vi "Sequencer Main - Copy.vi"() -> ()   [LabVIEW 2018] (continued)
                          n2869 = Array Subset(array=w5897, index=0, length=7) -> (w5898:string[])
                          n2870 = Bundle By Name(cluster=T15 {"Row"=0, "Column"=0} ("Active Cell:Active Cell"), "Row"=w5902, "Column"=5) -> (w5903:T15)
                          n2871 = Replace Array Subset(array=w5910, new element=w5898, index (row)=w5902) -> (w5909:string[][])  [unwired: 1 in]
                          n2872 = property on="Test Sequencer Run" class="MCListbox (strict)"("ItemNames"=w5909, "Value"=w5902, "ActiveCell"=w5903, "CellFontColor"=w5900) -> ()  [unwired: 2 in, 2 out]
                        }
                      }
                    }
                  }
                }
                frame #3 {
                  # "Test Steps Manager"
                  n2873 = in-place {
                    w5928 = 20
                    w5931 = 20
                    n2874 = global read "Global Variable.vi" "Current Step Nmb"() -> (w5935:u32)
                    n2875 = global read "Global Variable.vi" "Report Step Nmb"() -> (w5924:u32)
                    n2876 = Quotient & Remainder(x=w5935, y=w5931) -> (floor(x/y)=w5932:u32)  [unwired: 1 out]
                    n2877 = Quotient & Remainder(x=w5924, y=w5928) -> (floor(x/y)=w5927:u32)  [unwired: 1 out]
                    n2878 = Multiply(x=w5932, y=w5931) -> (x*y=w5930:u32)
                    n2879 = Multiply(x=w5927, y=w5928) -> (x*y=w5929:u32)
                    n2880 = Bundle By Name(cluster=T14 {"Row"=0, "Column"=0} ("Top Left Visible Cell"), "Row"=w5930) -> (w5934:T14)
                    n2881 = Bundle By Name(cluster=T14 {"Row"=0, "Column"=0} ("Top Left Visible Cell"), "Row"=w5929) -> (w5925:T14)
                    n2882 = property on="Test Sequencer" class="MCListbox (strict)"("TopLeft"=w5934) -> ()  [unwired: 2 in, 2 out]
                    n2883 = property on="Test Sequencer Run" class="MCListbox (strict)"("TopLeft"=w5925) -> ()  [unwired: 2 in, 2 out]
                  }
                  n2884 = global read "Global Variable.vi" "Current Step Nmb"() -> (w5920:u32)
                  n2885 = global read "Global Variable.vi" "Steps Nmb"() -> (w5921:u32)
                  n2886 = in-place {
                    n2887 = local read "Tab Edit/Run"() -> (w5936:enum32{"Edit", "Run"})
                    n2888 = case shown="\"Edit\", Default" w5936 {
                      frame "Edit", Default {
                        n2889 = case shown="True" "Delay 1S" {
                          frame False {
                          }
                          frame True {
                            n2890 = Wait (ms)(milliseconds to wait=u32 1000) -> ()  [unwired: 1 out]
                          }
                        }
                      }
                      frame "Run" {
                      }
                    }
                  }
                  n2891 = in-place {
                    # "Prevent False durring run in RUN windows"
                    n2892 = local read "Tab Edit/Run"() -> (w5922:enum32{"Edit", "Run"})
                    n2893 = case shown="\"Run\"" w5922 {
                      frame "Edit", Default {
                      }
                      frame "Run" {
                        n2894 = Wait (ms)(milliseconds to wait=u32 100) -> ()  [unwired: 1 out]
                      }
                    }
                  }
                  n2895 = Decrement(x=w5921) -> (x-1=w5919:u32)
                  n2896 = Equal?(x=w5919, y=w5920) -> (x = y?=w5918:bool)
                  n2897 = case shown="True" w5918 {
                    frame False {
                      n2898 = global write "Global Variable.vi" "System Status"(T1."Run Sequencer" ("System Status")) -> ()
                    }
                    frame True {
                      n2899 = global write "Global Variable.vi" "System Status"(T1."STOP Sequencer" ("System Status")) -> ()
                    }
                  }
                  n2900 = in-place {
                    n2901 = Tick Count (ms)() -> (millisecond timer value=w5939:u32)
                    n2902 = global write "Global Variable.vi" "Test Stop Time"(w5939) -> ()
                  }
                }
              }
            }
          }
        }
        frame "STOP Sequencer" {
          n2903 = in-place {
            in-place-border: w5943 -> [w5945]
            in-place-border: w5942 -> [w5944]
            n2904 = flat-sequence {
              tunnel: w5945 -> [w5993]
              tunnel: w5944 -> [w5992]
              frame #0 {
                n2905 = global read "Global Variable.vi" "Test Gen Status"() -> (w5946:bool)
                n2906 = in-place {
                  # "Create Log File"
                  n2907 = call "Ini_LogFile.vi"() -> ("error out"=w5948:errorcluster, "logFile Path"=w5949:refnum<file>)  [unwired: 10 in]
                  n2908 = global write "Global Variable.vi" "logFile Path"(w5949) -> ()
                  n2909 = local read "LogMsg"() -> (w5953:string)
                  n2910 = Write to Text File(file (use dialog)=w5949, text=w5953, error in=w5948) -> (refnum out=w5951:refnum<file>, error out=w5952:errorcluster)  [unwired: 1 in, 1 out]
                  n2911 = Close File(refnum=w5951, error in=w5952) -> (error out=w5950:errorcluster)  [unwired: 1 out]
                  n2912 = call <userlib>:"Clear All Errors__ogtk.vi"("Error In"=w5950) -> ()  [unwired: 3 in, 1 out]
                }
                n2913 = case shown="True" w5946 {
                  frame False {
                    w5964 = u32 16711680
                    n2914 = Bundle(w5964, w5964) -> (w5965:cluster{u32, u32})  [unwired: 1 in]
                    n2915 = Build Array(w5965) -> (w5966:cluster{u32, u32}[])
                    n2916 = property on="Gen Test Status" class="Bool (strict)"("Colors [4]"=w5966, "Value"=FALSE ("Gen Test Status"), "Strings [4]"=string[] ["FALSE", "PASS", "", ""]) -> ()  [unwired: 2 in, 2 out]
                  }
                  frame True {
                    w5969 = u32 40735
                    n2917 = Bundle(w5969, w5969) -> (w5967:cluster{u32, u32})  [unwired: 1 in]
                    n2918 = Build Array(w5967) -> (w5968:cluster{u32, u32}[])
                    n2919 = property on="Gen Test Status" class="Bool (strict)"("Colors [4]"=w5968, "Value"=TRUE ("Gen Test Status"), "Strings [4]"=string[] ["FALSE", "PASS", "", ""]) -> ()  [unwired: 2 in, 2 out]
                  }
                }
                n2920 = case shown="True" FALSE {
                  frame False {
                  }
                  frame True {
                    n2921 = One Button Dialog(message="STOP Sequencer") -> ()  [unwired: 1 in, 1 out]
                  }
                }
                n2922 = in-place {
                  in-place-border: w5946 -> [w5954]
                  n2923 = local read "Cnt Total"() -> (w5955:i32)
                  n2924 = case shown="True" w5954 {
                    frame False {
                      n2925 = local read "Cnt False"() -> (w5958:i32)
                      n2926 = Increment(x=w5958) -> (x+1=w5957:i32)
                      n2927 = local write "Cnt False"(w5957) -> ()
                    }
                    frame True {
                      n2928 = local read "Cnt Pass"() -> (w5960:i32)
                      n2929 = Increment(x=w5960) -> (x+1=w5959:i32)
                      n2930 = local write "Cnt Pass"(w5959) -> ()
                    }
                  }
                  n2931 = Increment(x=w5955) -> (x+1=w5956:i32)
                  n2932 = local write "Cnt Total"(w5956) -> ()
                }
              }
              frame #1 {
                w5974 = FALSE ("Enable Output")
                w5972 = 0.1 ("Current")
                w5973 = 0.0 ("Voltage")
                n2933 = global read "Global Variable.vi" "VISA Resource Name BK-9202"() -> (w5983:string)
                n2934 = call "bk9201 Set.vi"("Enable Output"=w5974, "Current"=w5972, "Voltage"=w5973, "VISA resource name"=w5983) -> ("error out"=w5979:errorcluster)  [unwired: 7 in]
                n2935 = local read "PowSupply - SET"() -> (w5976:T7)
                n2936 = local read "Switch Relay Modules"() -> (w5978:T5)
                n2937 = Bundle By Name(cluster=w5978, "Main Power Supplay ON/OFF"=w5974) -> (w5977:T5)
                n2938 = global read "Global Variable.vi" "Array Errors"() -> (w5981:errorcluster[])
                n2939 = Bundle By Name(cluster=w5976, "ON/OFF"=w5974, "Volt (V)"=w5973, "Current Limit (A)"=w5972) -> (w5975:T7)
                n2940 = global write "Global Variable.vi" "PowSupply ON/OFF"(w5974) -> ()
                n2941 = Replace Array Subset(array=w5981, new element=w5979, index=2) -> (w5982:errorcluster[])
                n2942 = local write "Switch Relay Modules"(w5977) -> ()
                n2943 = local write "PowSupply - SET"(w5975) -> ()
                n2944 = global write "Global Variable.vi" "Array Errors"(w5982) -> ()
              }
              frame #2 {
                n2945 = global read "Global Variable.vi" "COM Port RFID"() -> (w5987:refnum<visa-resource-name>)
                n2946 = call "Stop Reading.vi"("error in (no error)"=errorcluster {"status"=FALSE, "code"=0, "source"=""}, "Baud Rate"=u32 38400, "COM Port"=w5987) -> ("error out"=w5984:errorcluster)  [unwired: 6 in, 2 out]
                n2947 = call <userlib>:"Clear All Errors__ogtk.vi"("Error In"=w5984) -> ()  [unwired: 3 in, 1 out]
              }
              frame #3 {
                n2948 = call <vilib>:"Acquire Semaphore.vi"("error in (no error)"=w5993, "semaphore"=w5992) -> ("error out"=w5991:errorcluster, "semaphore out"=w5990:T13)  [unwired: 3 in, 1 out]
                n2949 = case shown="No Error" w5991 {
                  selector: w5991 -> [w6005 w6052]
                  tunnel: w5990 -> [w6004 w6051]
                  tunnel: [w6005 w6052] -> w5989
                  tunnel: [w6004 w6051] -> w5988
                  frame No Error {
                    w5999 = u8 1  # nCS
                    w6000 = T20 0 items=["Addr-0"=0, "Addr-1"=4, "Addr-2"=2, "Addr-3"=6, "Addr-4"=1, "Addr-5"=5, "Addr-6"=3, "Addr-7"=7] ("Addr")
                    w6010 = T20 7 items=["Addr-0"=0, "Addr-1"=4, "Addr-2"=2, "Addr-3"=6, "Addr-4"=1, "Addr-5"=5, "Addr-6"=3, "Addr-7"=7] ("Addr")
                    # "FALSE"
                    # "PASS"
                    # "nCS"
                    n2950 = global read "Global Variable.vi" "FTDI SPI Handle"() -> (w6001:u32)
                    n2951 = for {
                      N: 4 -> [_]
                      tunnel: w6001 -> [w6029]
                      tunnel: [w6021] -> w6011
                      i -> [w6024]
                      w6026 = u8 0  # nCS
                      w6025 = u16 0  # Channel Decimal
                      w6027 = TRUE  # Use Extra
                      n2952 = call "FTDI SPI GPIO Set.vi"("nCS"=w6026, "Mode"=T23."Set Decimal", "Use Extra"=w6027, "Channel Decimal"=w6025, "Addr"=w6024, "Handler In"=w6029) -> ("error out"=w6021:errorcluster, "LATCH Reg"=w6022:u16)  [unwired: 2 in, 2 out]
                      n2953 = Number To Boolean Array(number=w6022) -> (Boolean array=w6023:bool[])
                      n2954 = case shown="0" w6024 {
                        tunnel: w6023 -> [_ w6030 w6033 w6036 w6039 w6042 w6045 w6048]
                        frame -1, Default {
                        }
                        frame 0 {
                          n2955 = local read "Switch Relay Modules"() -> (w6032:T5)
                          n2956 = Bundle By Name(cluster=w6032, "SW 0"=w6030) -> (w6031:T5)
                          n2957 = local write "Switch Relay Modules"(w6031) -> ()
                        }
                        frame 1 {
                          n2958 = local read "Switch Relay Modules"() -> (w6035:T5)
                          n2959 = Bundle By Name(cluster=w6035, "SW 1"=w6033) -> (w6034:T5)
                          n2960 = local write "Switch Relay Modules"(w6034) -> ()
                        }
                        frame 2 {
                          n2961 = local read "Switch Relay Modules"() -> (w6038:T5)
                          n2962 = Bundle By Name(cluster=w6038, "SW 2"=w6036) -> (w6037:T5)
                          n2963 = local write "Switch Relay Modules"(w6037) -> ()
                        }
                        frame 3 {
                          n2964 = local read "Switch Relay Modules"() -> (w6041:T5)
                          n2965 = Bundle By Name(cluster=w6041, "SW 3"=w6039) -> (w6040:T5)
                          n2966 = local write "Switch Relay Modules"(w6040) -> ()
                        }
                        frame 4 {
                          n2967 = local read "Switch Relay Modules"() -> (w6044:T5)
                          n2968 = Bundle By Name(cluster=w6044, "SW 4"=w6042) -> (w6043:T5)
                          n2969 = local write "Switch Relay Modules"(w6043) -> ()
                        }
                        frame 5 {
                          n2970 = local read "Switch Relay Modules"() -> (w6047:T5)
                          n2971 = Bundle By Name(cluster=w6047, "SW 5"=w6045) -> (w6046:T5)
                          n2972 = local write "Switch Relay Modules"(w6046) -> ()
                        }
                        frame 6 {
                          n2973 = local read "Switch Relay Modules"() -> (w6050:T5)
                          n2974 = Bundle By Name(cluster=w6050, "SW 6"=w6048) -> (w6049:T5)
                          n2975 = local write "Switch Relay Modules"(w6049) -> ()
                        }
                      }
                    }
                    n2976 = local read "Gen Test Status"() -> (w5996:bool)
                    n2977 = global read "Global Variable.vi" "FTDI SPI Handle"() -> (w6016:u32)
                    n2978 = Select(t=1, s=w5996, f=2) -> (s? t:f=w5997:i32)
                    n2979 = call "FTDI SPI GPIO Set.vi"("nCS"=u8 2, "Mode"=T24."Set Decimal", "Use Extra"=TRUE, "Channel Decimal"=w5997, "Addr"=w6010, "Handler In"=w6016) -> ("error out"=w6012:errorcluster, "LATCH Reg"=w6009:u16)  [unwired: 2 in, 2 out]
                    n2980 = local read "Switch Relay Modules"() -> (w6007:T5)
                    n2981 = Number To Boolean Array(number=w6009) -> (Boolean array=w6008:bool[])
                    n2982 = Bundle By Name(cluster=w6007, "SW 7"=w6008) -> (w6006:T5)
                    n2983 = global read "Global Variable.vi" "Array Errors"() -> (w6019:errorcluster[])
                    n2984 = Merge Errors(w6011, w6012) -> (w6013:errorcluster)
                    n2985 = local write "Switch Relay Modules"(w6006) -> ()
                    n2986 = Replace Array Subset(array=w6019, new element=w6013, index=10) -> (w6020:errorcluster[])
                    n2987 = call "FTDI SPI GPIO Set.vi"("nCS"=w5999, "Use Extra"=TRUE, "Channel Decimal"=u16 0, "Addr"=w6000, "Handler In"=w6001) -> ()  [unwired: 3 in, 4 out]
                    n2988 = global write "Global Variable.vi" "Array Errors"(w6020) -> ()
                  }
                  frame Error {
                  }
                }
                n2989 = call <vilib>:"Release Semaphore.vi"("error in (no error)"=w5989, "semaphore"=w5988) -> ()  [unwired: 4 in, 2 out]
              }
              frame #4 {
                n2990 = local read "Restart Cnt"() -> (w6054:u16)
                n2991 = local read "Auto\nRestart"() -> (w6055:u16)
                n2992 = Less?(x=w6054, y=w6055) -> (x < y?=w6056:bool)
                n2993 = case shown="True" w6056 {
                  frame False {
                    n2994 = local read "Report Auto"() -> (w6060:bool)
                    n2995 = case shown="True" w6060 {
                      frame False {
                        n2996 = global write "Global Variable.vi" "System Status"(T1."Idle" ("System Status")) -> ()
                      }
                      frame True {
                        n2997 = global read "Global Variable.vi" "Retest Nmb"() -> (w6062:i16)
                        n2998 = case shown="0, Default" w6062 {
                          frame 0, Default {
                            n2999 = property on="Tab Control Main" class="TabCtl (strict)"("Value"=T2."Report" ("Tab Control Main")) -> ()  [unwired: 2 in, 2 out]
                            n3000 = global write "Global Variable.vi" "System Status"(T1."Report Generation" ("System Status")) -> ()
                          }
                          frame 1 {
                            n3001 = global write "Global Variable.vi" "Test Gen Status"(FALSE ("Test Gen Status")) -> ()
                            n3002 = global write "Global Variable.vi" "System Status"(T1."Idle" ("System Status")) -> ()
                          }
                        }
                      }
                    }
                    n3003 = local write "Auto\nRestart"(1) -> ()
                    n3004 = local write "Message"(">>>STOP SEQUENSER <<<") -> ()
                    n3005 = property on="Run Test" class="Bool"("DisabledEnum"=T18."Enabled" ("Disabled")) -> ()  [unwired: 2 in, 2 out]
                  }
                  frame True {
                    n3006 = local write "Auto\nReStart"(TRUE ("Auto\nReStart")) -> ()
                    n3007 = global write "Global Variable.vi" "Reset BARCODE"(TRUE ("Reset BARCODE")) -> ()
                    n3008 = local read "Report Auto"() -> (w6068:bool)
                    n3009 = case shown="False" w6068 {
                      frame False {
                        # "Idle"
                        n3010 = global write "Global Variable.vi" "System Status"(T1."Idle" ("System Status")) -> ()
                        n3011 = property on="Tab Control Main" class="TabCtl (strict)"("Value"=T2."TEST Board" ("Tab Control Main")) -> ()  [unwired: 2 in, 2 out]
                      }
                      frame True {
                        n3012 = global write "Global Variable.vi" "System Status"(T1."Report Generation" ("System Status")) -> ()
                        n3013 = property on="Tab Control Main" class="TabCtl (strict)"("Value"=T2."Report" ("Tab Control Main")) -> ()  [unwired: 2 in, 2 out]
                      }
                    }
                    n3014 = local write "Message"(">>> RESTART TEST Sequencer <<<") -> ()
                  }
                }
                n3015 = property on="Msg Str" class="Str"("Value"="STOP SEQUENSER\nReset ALL") -> ()  [unwired: 2 in, 2 out]
              }
            }
          }
        }
        frame "Report Generation" {
          n3016 = flat-sequence {
            tunnel: [w6089] -> w6082
            tunnel: [w6088] -> w6081
            tunnel: [w6085] -> w6080
            tunnel: [w6123] -> w6084
            tunnel: [w6122] -> w6083
            tunnel: w6082 -> [w6122]
            tunnel: w6081 -> [w6121]
            tunnel: w6080 -> [w6119]
            tunnel: w6084 -> [w6133]
            tunnel: [w6132] -> w6079
            tunnel: w6083 -> [w6132]
            tunnel: w6079 -> [w6140]
            tunnel: [w6141] -> w6078
            tunnel: [w6140] -> w6077
            tunnel: [w6138] -> w6076
            tunnel: [w6139] -> w6075
            tunnel: w6078 -> [w6180]
            tunnel: w6077 -> [w6179]
            tunnel: w6076 -> [w6177]
            tunnel: w6075 -> [w6178]
            frame #0 {
              w6086 = "<p>&nbsp;</p>" ("string")
              w6112 = u16 2 items=["Default", "US", "Metric"] ("measurement system (default)")
              # "table {\n  font-family: arial, sans-serif;\n  border-collapse: collapse;\n  width: 70%;\n}"
              # "Hardware Revision"
              n3017 = property on="Test Sequencer Run" class="MCListbox (strict)"() -> ("ColHdrString"=w6118:string[], "ItemNames"=w6114:string[][])  [unwired: 2 in, 2 out]
              n3018 = local read "Test Time"() -> (w6094:string)
              n3019 = call <vilib>:"New Report.vi"("report type"=T31."HTML") -> ("report out"=w6108:refnum<class "NI_report.lvclass">, "error out"=w6111:errorcluster)  [unwired: 5 in, 8 out]
              n3020 = local read "Customer"() -> (w6105:string)
              n3021 = local read "Under Test BOARD"() -> (w6104:string)
              n3022 = local read "Barcode"() -> (w6101:string)
              n3023 = property on="Operator" class="Ring (strict)"() -> ("RingText.Text"=w6100:string)  [unwired: 2 in, 2 out]
              n3024 = local read "Config"() -> (w6103:string)
              n3025 = global read "Global Variable.vi" "Report Step Nmb"() -> (w6091:u32)
              n3026 = call-dynamic "Set Report Margins.vi"("report in"=w6108, "margins (1.00)"=T32 {"top"=10.0, "left"=10.0, "right"=10.0, "bottom"=10.0}, "measurement system (default)"=w6112, "error in (no error)"=w6111) -> ("report out"=w6109:refnum<class "NI_report.lvclass">, "error out"=w6110:errorcluster)  [unwired: 9 in, 1 out]
              n3027 = local read "Gen Test Status"() -> (w6099:bool)
              n3028 = Array Subset(array=w6118, index=0, length=7) -> (w6115:string[])
              n3029 = Concatenate Strings("Measurement Results" ("Table Header"), "    (", "TestTime -" ("Table Header"), w6094, ")") -> (w6096:string)
              n3030 = Increment(x=w6091) -> (x+1=w6090:u32)
              n3031 = Build Array (concatenate)(w6115, w6114) -> (w6113:string[][])
              n3032 = call "html Header.vi"("Test Result"=w6099, "Test Operator"=w6100, "Company"=w6105, "Serial Numbe (SN)"=w6101, "Hardware Revision"="v1.1", "Product Info"=w6103, "Product Name"=w6104) -> ("html string"=w6087:string)  [unwired: 4 in]
              n3033 = call "html Table.vi"("Rows cnt"=w6090, "Table Header"=w6096, "In String Table"=w6113) -> ("html string out"=w6098:string)  [unwired: 8 in]
              n3034 = Concatenate Strings(w6087, w6086, w6098, w6086) -> (w6089:string)
              n3035 = call-dynamic "Append User Formatted HTML to Report.vi"("report in"=w6109, "HTML text"=w6089, "error in (no error)"=w6110) -> ("report out"=w6085:refnum<class "NI_report.lvclass">, "error out"=w6088:errorcluster)  [unwired: 11 out]
            }
            frame #1 {
              n3036 = in-place {
                in-place-border: w6119 -> [w6129]
                in-place-border: [w6128] -> w6123
                # "Local Temp File"
                n3037 = call <vilib>:"Application Directory.vi"() -> ("Application Directory"=w6131:path)
                n3038 = Build Path(base path=w6131, name or relative path="report.html") -> (appended path=w6128:path)
                n3039 = call-dynamic "Save Report to File.vi"("report in"=w6129, "report file path"=w6128) -> ()  [unwired: 12 in, 2 out]
                n3040 = Wait (ms)(milliseconds to wait=u32 250) -> ()  [unwired: 1 out]
              }
              n3041 = case shown="True" "Open in Default IE" {
                tunnel: w6121 -> [_ w6126]
                tunnel: w6119 -> [_ w6125]
                frame False {
                  n3042 = Wait (ms)(milliseconds to wait=u32 2000) -> ()  [unwired: 1 out]
                }
                frame True {
                  # "Open HTML Report in Browser VI"
                  n3043 = call-poly <vilib>:"Open HTML Report in Browser.vi"("report in"=w6125, "error in (no error)"=w6126) -> ()  [unwired: 14 out]
                }
              }
            }
            frame #2 {
              n3044 = Path To String(path=w6133) -> (string=w6136:string)
              n3045 = invoke class="IWebBrowser2" method="Navigate"(reference="WebBrowser", "URL"=w6136) -> (error out=w6134:errorcluster)  [unwired: 6 in, 7 out]
              n3046 = call <userlib>:"Clear All Errors__ogtk.vi"("Error In"=w6134) -> ()  [unwired: 3 in, 1 out]
            }
            frame #3 {
              # "Create BARCODE / Number FOLDER"
              n3047 = global read "Global Variable.vi" "DB Dir Path"() -> (w6137:path)
              n3048 = in-place {
                in-place-border: [w6159] -> w6139
                in-place-border: [w6146] -> w6138
                in-place-border: w6137 -> [w6144]
                # "Sub Dir?"
                # "FALSE Sub Dir?"
                n3049 = Get Date/Time String() -> (date string=w6154:string)  [unwired: 3 in, 1 out]
                n3050 = while {
                  shift-right: [w6170] -> w6155
                  shift-left: w6154 -> [w6173]
                  stop <- w6168 stop-if-true
                  # "Replase character / to _"
                  n3051 = call <vilib>:"Search and Replace Pattern.vi"("string"=w6173, "regular expression (\"\")"="/" ("substring (\"\")"), "replace string (\"\")"="_" ("replace string (\"\")")) -> ("result string"=w6170:string, "offset past match"=w6169:i32)  [unwired: 2 in]
                  n3052 = Less Than 0?(x=w6169) -> (x < 0?=w6168:bool)
                }
                n3053 = local read "Config"() -> (w6148:string)
                n3054 = Build Path(base path=w6144, name or relative path=w6155) -> (appended path=w6149:path)
                n3055 = Build Path(base path=w6149, name or relative path=w6148) -> (appended path=w6147:path)
                n3056 = call <vilib>:"Check if File or Folder Exists.vi"("path"=w6147) -> ("file or folder exists?"=w6153:bool, "dup path"=w6158:path)  [unwired: 8 in, 1 out]
                n3057 = Not(x=w6153) -> (.not. x?=w6157:bool)
                n3058 = case shown="True" w6157 {
                  tunnel: w6158 -> [w6164 w6167]
                  tunnel: [w6164 w6165] -> w6146
                  frame False {
                  }
                  frame True {
                    # "Time/Date Sub Dir"
                    n3059 = Create Folder(path (use dialog)=w6167) -> (created path=w6165:path, error out=w6166:errorcluster)  [unwired: 2 in, 1 out]
                    n3060 = call <userlib>:"Clear All Errors__ogtk.vi"("Error In"=w6166) -> ()  [unwired: 3 in, 1 out]
                  }
                }
                n3061 = Build Path(base path=w6146, name or relative path="FALSE") -> (appended path=w6151:path)
                n3062 = call <vilib>:"Check if File or Folder Exists.vi"("path"=w6151) -> ("file or folder exists?"=w6150:bool, "dup path"=w6145:path)  [unwired: 8 in, 1 out]
                n3063 = Not(x=w6150) -> (.not. x?=w6156:bool)
                n3064 = case shown="True" w6156 {
                  tunnel: w6145 -> [w6160 w6163]
                  tunnel: [w6160 w6161] -> w6159
                  frame False {
                  }
                  frame True {
                    # "FALSE Sub Dir"
                    n3065 = Create Folder(path (use dialog)=w6163) -> (created path=w6161:path, error out=w6162:errorcluster)  [unwired: 2 in, 1 out]
                    n3066 = call <userlib>:"Clear All Errors__ogtk.vi"("Error In"=w6162) -> ()  [unwired: 3 in, 1 out]
                  }
                }
              }
              n3067 = local read "Barcode"() -> (w6143:string)
              n3068 = in-place {
                in-place-border: w6143 -> [w6176]
                in-place-border: [w6174] -> w6141
                # "Length of Barcode > ?"
                n3069 = String Length(string=w6176) -> (length=w6175:i32)
                n3070 = Greater Than 0?(x=w6175) -> (x > 0?=w6174:bool)
              }
              n3071 = Wait (ms)(milliseconds to wait=u32 3000) -> ()  [unwired: 1 out]
            }
            frame #4 {
              # "Date"
              n3072 = case shown="True" w6180 {
                tunnel: w6179 -> [_ w6192]
                tunnel: w6178 -> [_ w6182]
                tunnel: w6177 -> [_ w6181]
                frame False {
                }
                frame True {
                  n3073 = call <vilib>:"New Report.vi"("report type"=T31."HTML") -> ("report out"=w6194:refnum<class "NI_report.lvclass">, "error out"=w6195:errorcluster)  [unwired: 5 in, 8 out]
                  n3074 = local read "Barcode"() -> (w6191:string)
                  n3075 = local read "Gen Test Status"() -> (w6187:bool)
                  n3076 = call-dynamic "Set Report Margins.vi"("report in"=w6194, "error in (no error)"=w6195) -> ("report out"=w6197:refnum<class "NI_report.lvclass">, "error out"=w6196:errorcluster)  [unwired: 11 in, 1 out]
                  n3077 = call-dynamic "Append User Formatted HTML to Report.vi"("report in"=w6197, "HTML text"=w6192, "error in (no error)"=w6196) -> ("report out"=w6184:refnum<class "NI_report.lvclass">, "error out"=w6193:errorcluster)  [unwired: 11 out]
                  n3078 = Concatenate Strings(w6191, ".html" ("string")) -> (w6185:string)
                  n3079 = Not(x=w6187) -> (.not. x?=w6186:bool)
                  n3080 = Build Path(base path=w6181, name or relative path=w6185) -> (appended path=w6188:path)
                  n3081 = call-dynamic "Save Report to File.vi"("report in"=w6184, "report file path"=w6188, "prompt to replace? (F)"=FALSE, "error in (no error)"=w6193) -> ("error out"=w6183:errorcluster)  [unwired: 10 in, 1 out]
                  n3082 = case shown="True" w6186 {
                    tunnel: w6182 -> [_ w6204]
                    tunnel: w6184 -> [_ w6202]
                    tunnel: w6185 -> [_ w6201]
                    frame False {
                    }
                    frame True {
                      n3083 = Build Path(base path=w6204, name or relative path=w6201) -> (appended path=w6203:path)
                      n3084 = call-dynamic "Save Report to File.vi"("report in"=w6202, "report file path"=w6203, "prompt to replace? (F)"=FALSE) -> ("error out"=w6199:errorcluster)  [unwired: 11 in, 1 out]
                      n3085 = call <userlib>:"Clear All Errors__ogtk.vi"("Error In"=w6199) -> ()  [unwired: 3 in, 1 out]
                    }
                  }
                  n3086 = call <userlib>:"Clear All Errors__ogtk.vi"("Error In"=w6183) -> ()  [unwired: 3 in, 1 out]
                }
              }
            }
            frame #5 {
              n3087 = in-place {
                n3088 = local read "Gen Test Status"() -> (w6207:bool)
                n3089 = local read "Cnt Total All"() -> (w6208:i32)
                n3090 = case shown="False" w6207 {
                  frame False {
                    n3091 = local read "Cnt False All"() -> (w6210:i32)
                    n3092 = Increment(x=w6210) -> (x+1=w6211:i32)
                    n3093 = local write "Cnt False All"(w6211) -> ()
                  }
                  frame True {
                    n3094 = local read "Cnt Pass All"() -> (w6212:i32)
                    n3095 = Increment(x=w6212) -> (x+1=w6213:i32)
                    n3096 = local write "Cnt Pass All"(w6213) -> ()
                  }
                }
                n3097 = Increment(x=w6208) -> (x+1=w6209:i32)
                n3098 = local write "Cnt Total All"(w6209) -> ()
              }
              n3099 = global write "Global Variable.vi" "System Status"(T1."Idle" ("System Status")) -> ()
              n3100 = property on="Tab Control Main" class="TabCtl (strict)"("Value"=T2."TEST Board" ("Tab Control Main")) -> ()  [unwired: 2 in, 2 out]
            }
            frame #6 {
              n3101 = local read "System INI Config File"() -> (w6214:path)
              n3102 = in-place {
                in-place-border: w6214 -> [w6226]
                w6227 = "REPORT"
                # "Write DATA To INI Sys File"
                n3103 = local read "Cnt Total All"() -> (w6222:i32)
                n3104 = call <vilib>:"Open Config Data.vi"("configuration file path"=w6226) -> ("error out"=w6224:errorcluster, "refnum"=w6225:T19)  [unwired: 8 in, 1 out]
                n3105 = local read "Cnt Pass All"() -> (w6215:i32)
                n3106 = call-poly <vilib>:"Write Key.vi"("section"=w6227, "error in (no error)"=w6224, "value"=w6222, "key"="TOTAL", "refnum"=w6225) -> ("error out"=w6228:errorcluster, "refnum out"=w6231:T19)  [unwired: 4 in, 1 out]
                n3107 = local read "Cnt False All"() -> (w6216:i32)
                n3108 = call-poly <vilib>:"Write Key.vi"("section"=w6227, "error in (no error)"=w6228, "value"=w6215, "key"="PASS", "refnum"=w6231) -> ("error out"=w6229:errorcluster, "refnum out"=w6230:T19)  [unwired: 4 in, 1 out]
                n3109 = call-poly <vilib>:"Write Key.vi"("section"=w6227, "error in (no error)"=w6229, "value"=w6216, "key"="FALSE", "refnum"=w6230) -> ("error out"=w6218:errorcluster, "refnum out"=w6219:T19)  [unwired: 4 in, 1 out]
                n3110 = call <vilib>:"Close Config Data.vi"("error in (no error)"=w6218, "refnum"=w6219) -> ("error out"=w6217:errorcluster)  [unwired: 8 in, 1 out]
                n3111 = call <vilib>:"Simple Error Handler.vi"("error in (no error)"=w6217) -> ()  [unwired: 4 in, 5 out]
              }
            }
          }
        }
        frame "QUIT" {
        }
        frame "Test Load Monitor" {
          n3112 = global write "Global Variable.vi" "System Status"(T1."Idle" ("System Status")) -> ()
        }
      }
    }
  }
